vi "Divider1.vi"() -> (8 "Divider1":refnum<class "Divider1.lvclass">)   [LabVIEW 2017, in "Divider1.lvclass"]
uses:
  Divider1.lvclass
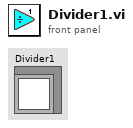
[diagram p1: front panel]
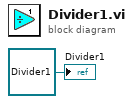
[diagram p0: block diagram]
diagram:
  "Divider1" <- refnum<class "Divider1.lvclass"> refnum ("Divider1.lvclass")
